vi "YAG_init.v3.vi"(8 "error in (no error)":errorcluster, 9 "initial V":dbl=700.0, 10 "initial rep rate":dbl=10.0, 11 "VISA Refnum in":refnum<visa-resource-name>="COM1") -> (0 "error out":errorcluster={"status"=FALSE, "code"=1073676294, "source"="VISA Read in Cmd-Reply.vi->YAG_init.vi->YAG_Control.v2.vi"}, 3 "VISA Refnum out":refnum<visa-resource-name>="COM1")   [LabVIEW 2018]
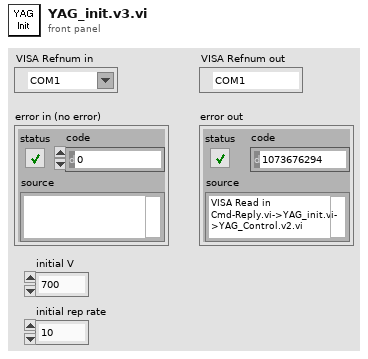
[diagram p1: front panel]
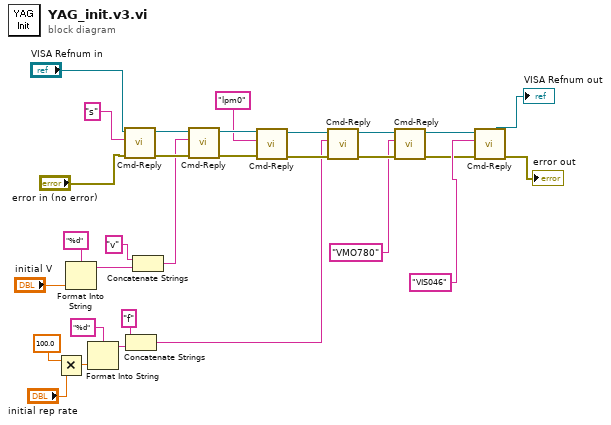
[diagram p0: block diagram]
diagram:
  n1 = Multiply(x=100.0, y="initial rep rate") -> (x*y=w16:dbl)
  n2 = Format Into String(format string="%d", "initial V") -> (resulting string=w22:string)  [unwired: 2 in, 1 out]
  n3 = Format Into String(format string="%d", w16) -> (resulting string=w14:string)  [unwired: 2 in, 1 out]
  n4 = call "Cmd-Reply.vi"("error in (no error)"="error in (no error)", "cmd"="s", "VISA Refnum in"="VISA Refnum in") -> ("error out"=w27:errorcluster, "VISA Refnum out"=w25:refnum<visa-resource-name>)  [unwired: 6 in, 1 out]
  n5 = Concatenate Strings("f" ("string"), w14) -> (w9:string)
  n6 = Concatenate Strings("v" ("string"), w22) -> (w19:string)
  n7 = call "Cmd-Reply.vi"("error in (no error)"=w27, "cmd"=w19, "VISA Refnum in"=w25) -> ("error out"=w26:errorcluster, "VISA Refnum out"=w24:refnum<visa-resource-name>)  [unwired: 6 in, 1 out]
  n8 = call "Cmd-Reply.vi"("error in (no error)"=w26, "cmd"="lpm0", "VISA Refnum in"=w24) -> ("error out"=w11:errorcluster, "VISA Refnum out"=w12:refnum<visa-resource-name>)  [unwired: 6 in, 1 out]
  n9 = call "Cmd-Reply.vi"("error in (no error)"=w11, "cmd"=w9, "VISA Refnum in"=w12) -> ("error out"=w4:errorcluster, "VISA Refnum out"=w5:refnum<visa-resource-name>)  [unwired: 6 in, 1 out]
  n10 = call "Cmd-Reply.vi"("error in (no error)"=w4, "cmd"="VMO780" ("concatenated string"), "VISA Refnum in"=w5) -> ("error out"=w1:errorcluster, "VISA Refnum out"=w6:refnum<visa-resource-name>)  [unwired: 6 in, 1 out]
  n11 = call "Cmd-Reply.vi"("error in (no error)"=w1, "cmd"="VIS046" ("concatenated string"), "VISA Refnum in"=w6) -> ("error out"=→"error out":errorcluster, "VISA Refnum out"=→"VISA Refnum out":refnum<visa-resource-name>)  [unwired: 6 in, 1 out]
